vi "HookedMessage.vi"() -> (1 "Hook":string="[XnSM*hook]", 2 "Hooked Message":T1={"Hook"="[XnSM*hook]", "Length"=0, "Reply?"=FALSE, "Data"=""})   [LabVIEW 2010]
uses:
  XStateMessage.ctl
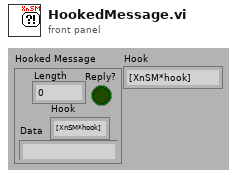
[diagram p1: front panel]
types:
  T1 = typedef "XStateMessage.ctl" = cluster{"Hook":string, "Length":u16, "Reply?":bool, "Data":string}
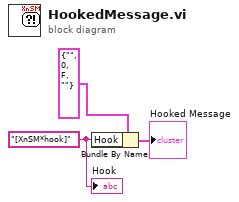
[diagram p0: block diagram]
diagram:
  w1 = "[XnSM*hook]" ("Hook")
  n1 = Bundle By Name(cluster=T1 {"Hook"="", "Length"=0, "Reply?"=FALSE, "Data"=""} ("XStateMessage"), "Hook"=w1) -> (→"Hooked Message":T1)
  "Hook" <- w1
